vi "Configure Simulator.vi"(6 "Obstacle Radius":dbl, 7 "LIDAR Characteristics":T2, 8 "error in (no error)":errorcluster, 9 "Initial Vehicle Pose":T1={"Initial Location"={"x"=0.0, "y"=0.0}, "Initial Heading"=45.0, "Initial Location ( GPS )"={"Latitude"=0.0, "Longitude"=0.0}}, 10 "Obstacle Locations":cluster{"x":dbl, "y":dbl}[](array[cluster]), 11 "Simulator in":refnum<class "Simulator.lvclass">) -> (0 "error out":errorcluster, 3 "Simulator out":refnum<class "Simulator.lvclass">)   [LabVIEW 2011, in "Simulator.lvclass"]
uses:
  Simulator.lvclass
  Simulator.lvclass/Simulator.ctl
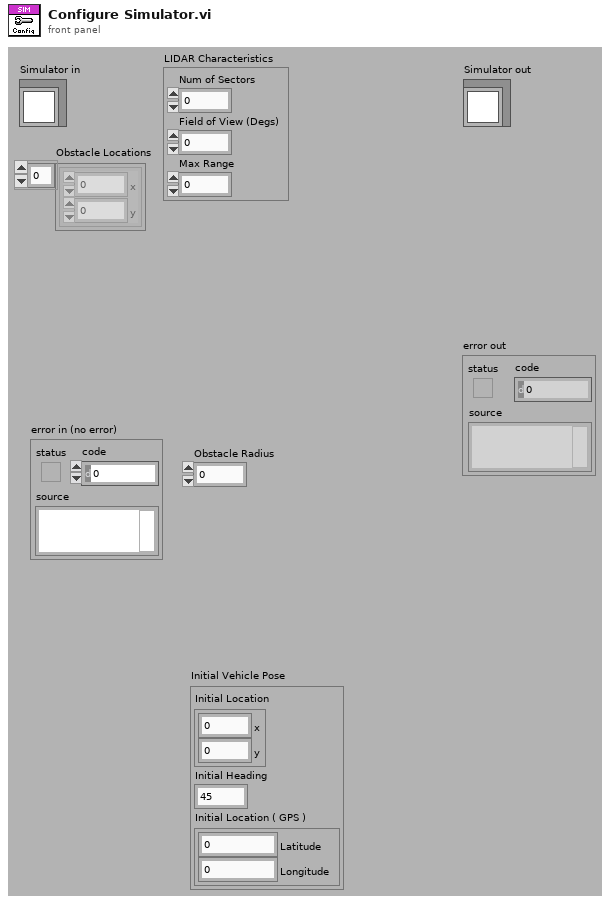
[diagram p1: front panel]
types:
  T1 = cluster{"Initial Location":cluster{"x":dbl, "y":dbl}, "Initial Heading":dbl, "Initial Location ( GPS )":cluster{"Latitude":dbl, "Longitude":dbl}}
  T2 = cluster{"Num of Sectors":i32, "Field of View (Degs)":dbl, "Max Range":dbl}
  T3 = cluster{"Num of Sectors":i32, "Field of View":dbl, "Max Range":dbl, "Rads per Sector":dbl}
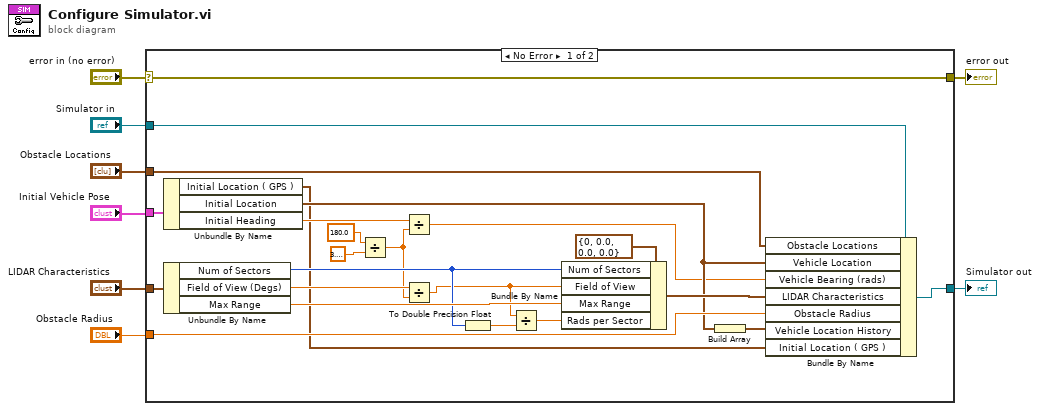
[diagram p0: block diagram]
diagram:
  n1 = case shown="No Error" "error in (no error)" {
    selector: "error in (no error)" -> [w30 w33]
    tunnel: [w30 w33] -> w7
    tunnel: [w29 w32] -> w5
    tunnel: "Simulator in" -> [w31 w32]
    tunnel: "Obstacle Locations" -> [w28 _]
    tunnel: "LIDAR Characteristics" -> [w27 _]
    tunnel: "Obstacle Radius" -> [w20 _]
    tunnel: "Initial Vehicle Pose" -> [w19 _]
    frame No Error {
      n2 = Unbundle By Name(w19) -> ("Initial Location ( GPS )"=w9:cluster{"Latitude":dbl, "Longitude":dbl}, "Initial Location"=w17:cluster{"x":dbl, "y":dbl}, "Initial Heading"=w12:dbl)
      n3 = Unbundle By Name(w27) -> ("Num of Sectors"=w23:i32, "Field of View (Degs)"=w16:dbl, "Max Range"=w25:dbl)
      n4 = Divide(x=180.0 ("y"), y=3.141592653589793) -> (x/y=w11:dbl)
      n5 = Divide(x=w12, y=w11) -> (x/y=w10:dbl)
      n6 = Divide(x=w16, y=w11) -> (x/y=w15:dbl)
      n7 = To Double Precision Float(number=w23) -> (double precision float=w22:dbl)
      n8 = Divide(x=w15, y=w22) -> (x/y=w21:dbl)
      n9 = Bundle By Name(cluster=T3 {"Num of Sectors"=0, "Field of View"=0.0, "Max Range"=0.0, "Rads per Sector"=0.0} ("LIDAR Characteristics"), "Num of Sectors"=w23, "Field of View"=w15, "Max Range"=w25, "Rads per Sector"=w21) -> (w24:T3)
      n10 = Build Array(w17) -> (w18:cluster{"x":dbl, "y":dbl}[])
      n11 = Bundle By Name(cluster=w31, "Obstacle Locations"=w28, "Vehicle Location"=w17, "Vehicle Bearing (rads)"=w10, "LIDAR Characteristics"=w24, "Obstacle Radius"=w20, "Vehicle Location History"=w18, "Initial Location ( GPS )"=w9) -> (w29:refnum<class "Simulator.lvclass">)
    }
    frame Error {
    }
  }
  "error out" <- w7
  "Simulator out" <- w5
